vi "Hyperspectral Camera Configuration.vi"(8 "error in":errorcluster, 11 "Camera Session":T1) -> (0 "error out":errorcluster, 3 "Camera Session out":T1)   [LabVIEW 2023]
doc: "Configure hyperspectral camera with verified parameters."
uses:
  <resource>/objmgr/imaqdx.rc
  <vilib>/userDefined/High Color/IMAQdx.ctl
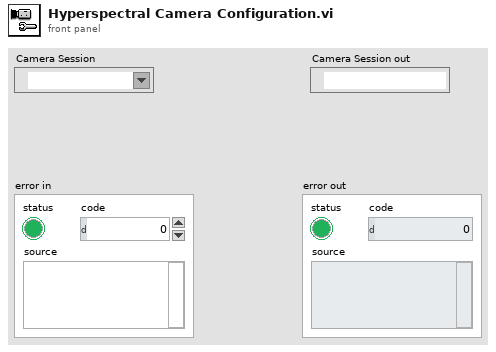
[diagram p1: front panel]
types:
  T1 = typedef "IMAQdx.ctl" = refnum<k21>
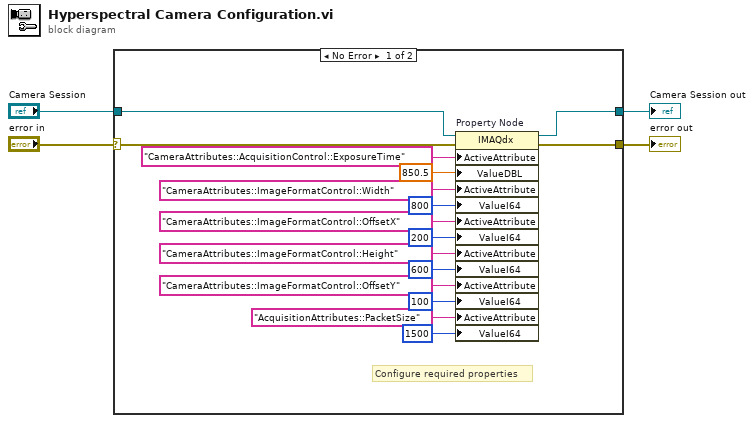
[diagram p0: block diagram]
diagram:
  n1 = case shown="No Error" "error in" {
    selector: "error in" -> [w7 w22]
    tunnel: "Camera Session" -> [w8 w21]
    tunnel: [w6 w21] -> w2
    tunnel: [w5 w22] -> w1
    frame No Error {
      # "Configure required properties"
      n2 = property on="Property Node" class="IMAQdx"(reference=w8, error in=w7, "ActiveAttribute"="CameraAttributes::AcquisitionControl::ExposureTime", "ValueDBL"=850.5 ("ExposureTime (ms)"), "ActiveAttribute"="CameraAttributes::ImageFormatControl::Width", "ValueI64"=i64 800 ("Width"), "ActiveAttribute"="CameraAttributes::ImageFormatControl::OffsetX", "ValueI64"=i64 200 ("OffsetX"), "ActiveAttribute"="CameraAttributes::ImageFormatControl::Height", "ValueI64"=i64 600 ("Height"), "ActiveAttribute"="CameraAttributes::ImageFormatControl::OffsetY", "ValueI64"=i64 100 ("OffsetY"), "ActiveAttribute"="AcquisitionAttributes::PacketSize", "ValueI64"=i64 1500 ("Packet size")) -> (reference out=w6:T1, error out=w5:errorcluster)
    }
    frame Error {
    }
  }
  "Camera Session out" <- w2
  "error out" <- w1
